vi "Jeffress_model_v006.vi"() -> ()   [LabVIEW 2019]
panel:
  out "Index":string
  out "new picture":picture
  in  "stop":bool
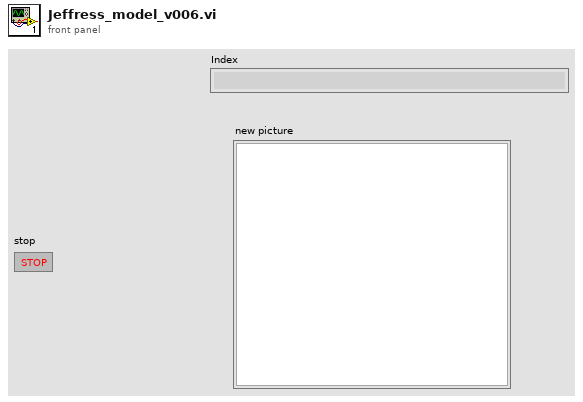
[diagram p1: front panel]
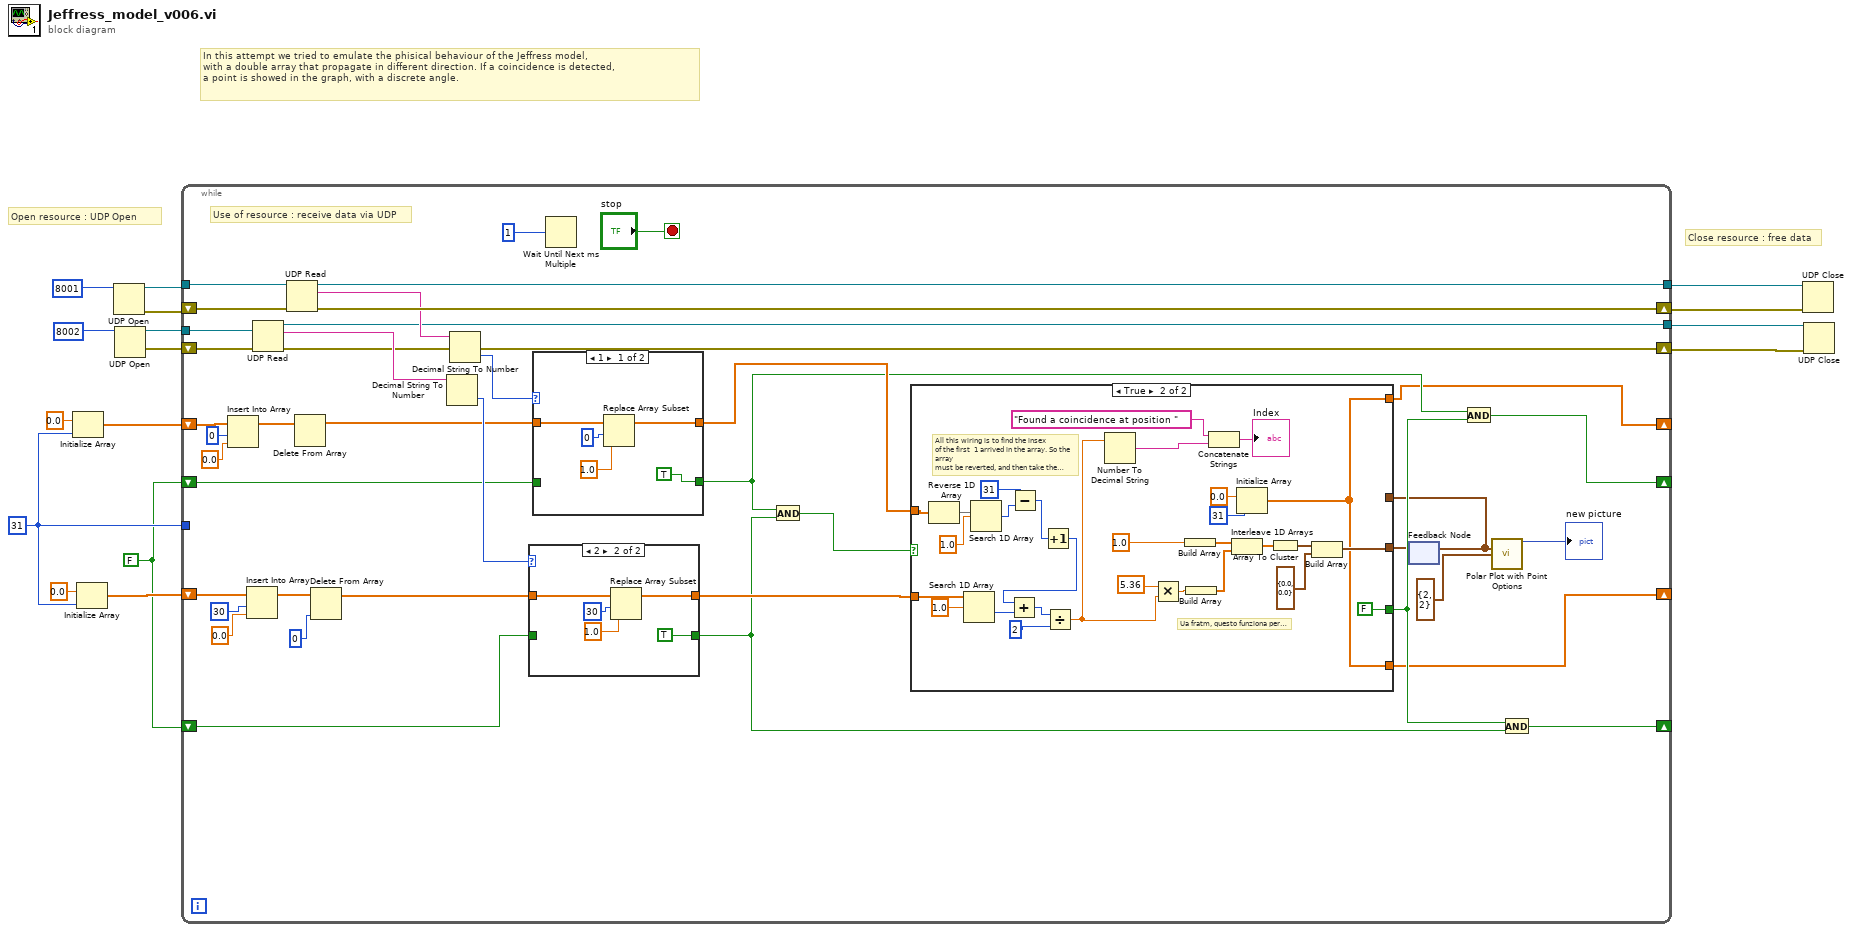
[diagram p0: block diagram]
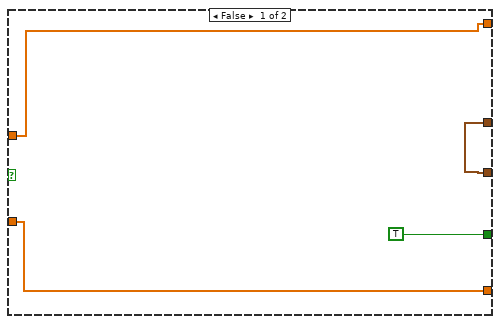
[diagram p2: hidden frame]
diagram:
  w1 = FALSE
  w2 = 31 ("dimension size")
  # "In this attempt we tried to emulate the phisical behaviour of the Jeffress model,\nwith a double array that propagate in different direction. If a coincidence is detected,\na point is showed in the graph, with a discrete angle."
  # "Close resource : free data"
  # "Open resource : UDP Open"
  n1 = Initialize Array(0.0 ("element"), w2) -> (w5:dbl[])
  n2 = Initialize Array(0.0 ("element"), w2) -> (w3:dbl[])
  n3 = UDP Open(11:u16 8001) -> (port=w14:refnum<k16>, 0:w16:errorcluster)  [unwired: 4 in, 1 out]
  n4 = UDP Open(11:u16 8002) -> (port=w10:refnum<k16>, 0:w9:errorcluster)  [unwired: 4 in, 1 out]
  n5 = while {
    tunnel: w14 -> [w53]
    tunnel: [w52] -> w13
    shift-right: [w55] -> w15
    shift-left: w16 -> [w54]
    tunnel: w10 -> [w46]
    shift-right: [w42] -> w8
    shift-left: w9 -> [w45]
    tunnel: [w43] -> w7
    shift-right: [w20] -> _
    shift-left: w5 -> [w41]
    shift-right: [w19] -> _
    shift-left: w3 -> [w33]
    tunnel: w2 -> [_]
    shift-right: [w22] -> _
    shift-left: w1 -> [w27]
    shift-right: [w21] -> _
    shift-left: w1 -> [w26]
    stop <- "stop" stop-if-true
    # "Use of resource : receive data via UDP"
    n6 = Insert Into Array(array=w41, index=0, new element=0.0 ("new element/subarray")) -> (w38:dbl[])
    n7 = Insert Into Array(array=w33, index=30, new element=0.0 ("new element/subarray")) -> (w34:dbl[])
    n8 = UDP Read(connection ID=w46, 8:w45) -> (data out=w47:string, error out=w42:errorcluster, 3:w43:refnum<k16>)  [unwired: 2 in, 2 out]
    n9 = UDP Read(connection ID=w53, 8:w54) -> (data out=w48:string, error out=w55:errorcluster, 3:w52:refnum<k16>)  [unwired: 2 in, 2 out]
    n10 = Delete From Array(array=w38) -> (array with subset deleted=w37:dbl[])  [unwired: 2 in, 1 out]
    n11 = Delete From Array(array=w34, index=0) -> (array with subset deleted=w31:dbl[])  [unwired: 1 in, 1 out]
    n12 = Decimal String To Number(string=w47) -> (number=w44:i32)  [unwired: 2 in, 1 out]
    n13 = Decimal String To Number(string=w48) -> (number=w49:i32)  [unwired: 2 in, 1 out]
    n14 = case shown="2" w44 {
      tunnel: [w92 w95] -> w28
      tunnel: w31 -> [w92 w94]
      tunnel: [w91 TRUE] -> w25
      tunnel: w26 -> [w91 _]
      frame Default {
      }
      frame 2 {
        n15 = Replace Array Subset(array=w94, new element=1.0 ("new element/subarray"), index=30) -> (w95:dbl[])
      }
    }
    n16 = case shown="1" w49 {
      tunnel: [w100 w104] -> w29
      tunnel: w37 -> [w99 w104]
      tunnel: [TRUE w103] -> w23
      tunnel: w27 -> [_ w103]
      frame 1 {
        n17 = Replace Array Subset(array=w99, new element=1.0 ("new element/subarray"), index=0) -> (w100:dbl[])
      }
      frame Default {
      }
    }
    n18 = Wait Until Next ms Multiple(millisecond multiple=u32 1) -> ()  [unwired: 1 out]
    n19 = And(x=w23, y=w25) -> (x .and. y?=w30:bool)
    n20 = feedback #1() -> (w17:cluster{"[0]":dbl, "[1]":dbl}[])  [unwired: 1 in]
    n21 = case shown="True" w30 {
      tunnel: [w58 w66] -> w18
      tunnel: w29 -> [w60 w79]
      tunnel: w28 -> [w59 w86]
      tunnel: [TRUE FALSE] -> w24
      tunnel: [w60 w62] -> w20
      tunnel: [w59 w62] -> w19
      tunnel: w17 -> [w58 _]
      frame False {
      }
      frame True {
        # "Ua fratm, questo funziona per forza"
        # "All this wiring is to find the insex\nof the first  1 arrived in the array. So the array \nmust be reverted, and then take the original \nindex."
        n22 = Reverse 1D Array(array=w79) -> (reversed array=w78:dbl[])
        n23 = Search 1D Array(1D array=w86, element=1.0) -> (index of element=w84:i32)  [unwired: 1 in]
        n24 = Search 1D Array(1D array=w78, element=1.0) -> (index of element=w74:i32)  [unwired: 1 in]
        n25 = Subtract(x=31, y=w74) -> (x-y=w72:i32)
        n26 = Increment(x=w72) -> (x+1=w71:i32)
        n27 = Add(x=w71, y=w84) -> (x+y=w83:i32)
        n28 = Divide(x=w83, y=2) -> (x/y=w80:dbl)
        n29 = Number To Decimal String(number=w80) -> (decimal integer string=w89:string)  [unwired: 1 in]
        n30 = Multiply(x=5.36, y=w80) -> (x*y=w90:dbl)
        n31 = Build Array(1.0) -> (w70:dbl[])
        n32 = Build Array(w90) -> (w69:dbl[])
        n33 = Concatenate Strings("Found a coincidence at position ", w89) -> (→"Index":string)
        n34 = Interleave 1D Arrays(w70, w69) -> (w68:dbl[])
        n35 = Initialize Array(0.0 ("element"), 31 ("dimension size")) -> (w62:dbl[])
        n36 = Array To Cluster(array=w68) -> (cluster=w67:cluster{"[0]":dbl, "[1]":dbl})
        n37 = Build Array(w67, cluster{"[0]":dbl, "[1]":dbl} {"[0]"=0.0, "[1]"=0.0} ("element")) -> (w66:cluster{"[0]":dbl, "[1]":dbl}[])
      }
    }
    n38 = feedback-in #1(w18) -> ()
    n39 = And(x=w23, y=w24) -> (x .and. y?=w22:bool)
    n40 = call <vilib>:"Polar Plot with Point Options.vi"("data array [mag, phase (deg)]"=w17, "top left point(0, 0)"=cluster{"x":i16, "y":i16} {"x"=2, "y"=2}) -> ("new picture"=→"new picture":picture)  [unwired: 13 in]
    n41 = And(x=w24, y=w25) -> (x .and. y?=w21:bool)
  }
  n42 = UDP Close(connection ID=w13, 8:w15) -> ()  [unwired: 2 out]
  n43 = UDP Close(connection ID=w7, 8:w8) -> ()  [unwired: 2 out]
